vi "Read Clone name.vi"(8 "error in (no error)":errorcluster, 11 "Fiber Auto Collimation panel in":refnum<class "Fiber Auto Collimation panel.lvclass">) -> (0 "error out":errorcluster, 2 "Clone name":string, 3 "Fiber Auto Collimation panel out":refnum<class "Fiber Auto Collimation panel.lvclass">)   [LabVIEW 2018, in "Fiber Auto Collimation panel.lvclass"]
doc: "The \"Clone name\" is only needed if this is a Panel class that can be open more than once. If the panel will only be open once at a time, don't bother using this element of the private data for anything.\n\nIf the panel can be open more than once simultaneously, just be sure that each instance of the panel has a unique non-blank name.\n\nNote that all clone names will be in lower case and will have been trimmed to remove whitespace on the ends."
uses:
  Fiber Auto Collimation panel.lvclass
  Fiber Auto Collimation panel.lvclass/Fiber Auto Collimation panel.ctl
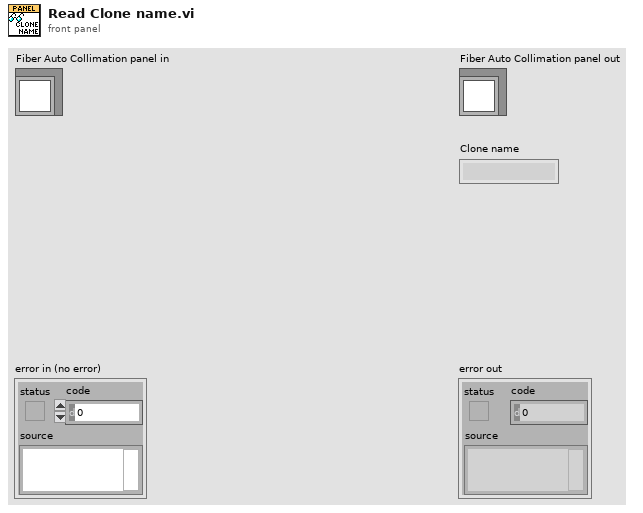
[diagram p1: front panel]
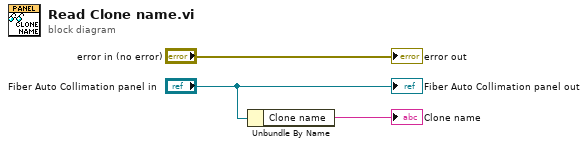
[diagram p0: block diagram]
diagram:
  n1 = Unbundle By Name("Fiber Auto Collimation panel in") -> ("Clone name"=→"Clone name":string)
  "error out" <- "error in (no error)"
  "Fiber Auto Collimation panel out" <- "Fiber Auto Collimation panel in"
